vi "Sort TaskView.vi"(8 "error in (no error)":errorcluster, 10 "Clicked Column":i32, 11 "BuildServer in":refnum<class "BuildServer.lvclass">) -> (0 "error out":errorcluster, 3 "BuildServer out":refnum<class "BuildServer.lvclass">)   [LabVIEW 2017, in "BuildServer.lvlib" / "BuildServer.lvclass"]
uses:
  BuildServer.lvclass
  BuildServer.lvclass/BuildServer.ctl
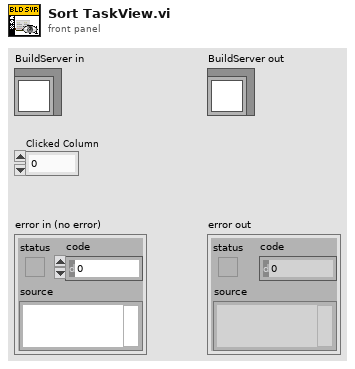
[diagram p1: front panel]
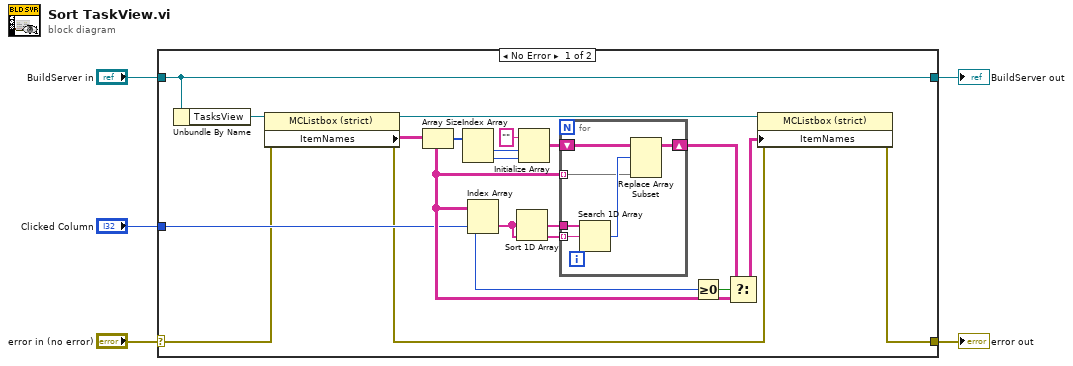
[diagram p0: block diagram]
diagram:
  n1 = case shown="No Error" "error in (no error)" {
    selector: "error in (no error)" -> [w8 w31]
    tunnel: [w7 w31] -> w4
    tunnel: [w10 w30] -> w2
    tunnel: "BuildServer in" -> [w10 w30]
    tunnel: "Clicked Column" -> [w11 _]
    frame No Error {
      n2 = Unbundle By Name(w10) -> ("TasksView"=w9:refnum<vi>)
      n3 = property on="Property Node" class="MCListbox (strict)"(reference=w9, error in=w8) -> (reference out=w12:refnum<vi>, error out=w6:errorcluster, "ItemNames"=w13:string[][])
      n4 = Array Size(array=w13) -> (size(s)=w20:i32[])
      n5 = Index Array(array=w20) -> (element #1=w19:i32, element #2=w18:i32)  [unwired: 2 in]
      n6 = Index Array(array=w13, index (col)=w11) -> (element=w22:string[])  [unwired: 1 in]
      n7 = Sort 1D Array(array=w22) -> (sorted array=w23:string[])
      n8 = Initialize Array("", w19, w18) -> (w17:string[][])
      n9 = for {
        tunnel: w13 -> [w25] mode=indexing
        shift-right: [w24] -> w15
        shift-left: w17 -> [w27]
        tunnel: w23 -> [w29]
        tunnel: w22 -> [w28] mode=indexing
        n10 = Search 1D Array(1D array=w29, element=w28) -> (index of element=w26:i32)  [unwired: 1 in]
        n11 = Replace Array Subset(array=w27, new element=w25, index (row)=w26) -> (w24:string[][])  [unwired: 1 in]
      }
      n12 = Greater Or Equal To 0?(x=w11) -> (x >= 0?=w16:bool)
      n13 = Select(t=w15, s=w16, f=w13) -> (s? t:f=w14:string[][])
      n14 = property on="Property Node" class="MCListbox (strict)"(reference=w12, error in=w6, "ItemNames"=w14) -> (error out=w7:errorcluster)  [unwired: 1 out]
    }
    frame Error {
    }
  }
  "error out" <- w4
  "BuildServer out" <- w2
